vi "Matches.vi"(8 "error in (no error)":errorcluster, 10 "Actual":variant, 11 "ErrorMessageContains in":refnum<class "ErrorMessageContains.lvclass">) -> (0 "error out":errorcluster, 2 "Result":bool, 3 "ErrorMessageContains out":refnum<class "ErrorMessageContains.lvclass">)   [LabVIEW 2017, in "Transparent Assertions.lvlib" / "ErrorMessageContains.lvclass"]
doc: "Evaluates the constraint for <B>Actual</B>. Returns true if the constraint is met."
uses:
  ErrorMessageContains.lvclass
  ErrorMessageContains.lvclass/ErrorMessageContains.ctl
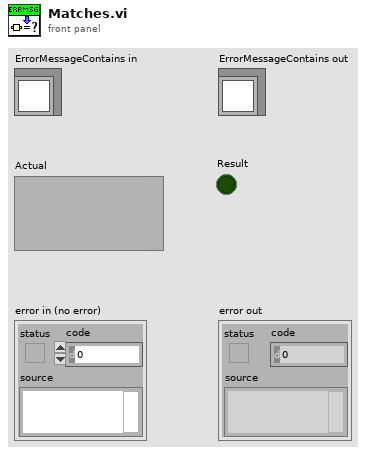
[diagram p1: front panel]
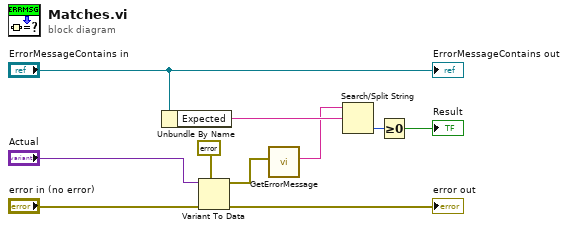
[diagram p0: block diagram]
diagram:
  n1 = Unbundle By Name("ErrorMessageContains in") -> ("Expected"=w9:string)
  n2 = Variant To Data(error in="error in (no error)", type=errorcluster {"status"=FALSE, "code"=0, "source"=""}, Variant="Actual") -> (data=w3:errorcluster, error out=→"error out":errorcluster)
  n3 = call "GetErrorMessage.vi"("error in (no error)"=w3) -> ("Error Message"=w2:string)  [unwired: 10 in]
  n4 = Search/Split String(string=w2, search string/char (-)=w9) -> (offset of match=w8:i32)  [unwired: 1 in, 2 out]
  n5 = Greater Or Equal To 0?(x=w8) -> (x >= 0?=→"Result":bool)
  "ErrorMessageContains out" <- "ErrorMessageContains in"
